vi "Simple Reader.vi"(8 "error in (no error)":errorcluster, 11 "Cryo-Con Driver in":refnum<class "Cryo-Con Driver.lvclass">) -> (0 "error out":errorcluster, 2 "Signals":dbl[](array[numeric]), 3 "Cryo-Con Driver out":refnum<class "Cryo-Con Driver.lvclass">)   [LabVIEW 2019, in "Cryo-Con Driver.lvclass"]
uses:
  Cryo-Con Driver.lvclass
  C:/GitHub/NHMFL_Core/Libraries/Instruments/VISA Instrument/VISA Instrument.lvclass
  C:/GitHub/NHMFL_Core/Libraries/Instruments/Temperature Controller Driver/Temperature Controller Driver.lvclass
  VISA Instrument/VISA Instrument.lvclass/VISA Instrument.ctl
  VISA Instrument/Read VISA resource.vi
  VISA Instrument/Write VISA resource.vi
  Temperature Controller Driver/Read T controller configuration.vi
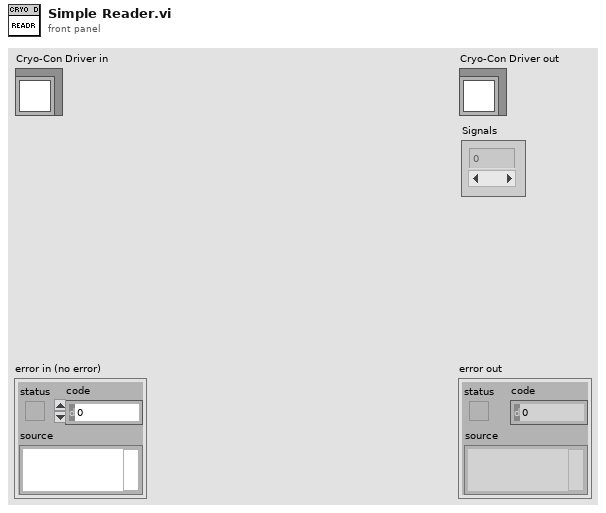
[diagram p1: front panel]
types:
  T1 = typedef "T controller configuration.ctl" = cluster{"Record Channels":string[], "Add raw signal":bool, "New set point":dbl, "Record heater":bool}
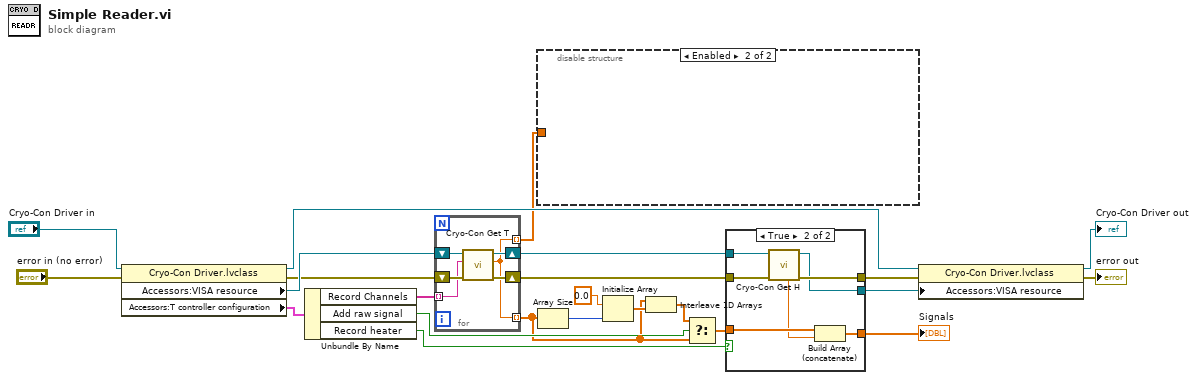
[diagram p0: block diagram]
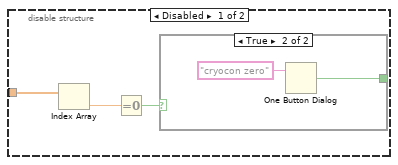
[diagram p2: hidden frame]
diagram:
  n1 = property class="Cryo-Con Driver.lvclass"(reference="Cryo-Con Driver in", error in="error in (no error)") -> (reference out=w17:refnum<class "Cryo-Con Driver.lvclass">, error out=w19:errorcluster, "Accessors:VISA resource"=w20:refnum<visa-resource-name>, "Accessors:T controller configuration"=w21:T1)
  n2 = Unbundle By Name(w21) -> ("Record Channels"=w22:string[], "Add raw signal"=w12:bool, "Record heater"=w4:bool)
  n3 = for {
    tunnel: w22 -> [w25] mode=indexing
    tunnel: [w24] -> w9 mode=indexing
    shift-right: [w27] -> w8
    shift-left: w19 -> [w28]
    shift-right: [w26] -> w7
    shift-left: w20 -> [w29]
    tunnel: [w24] -> w1 mode=indexing
    n4 = call "Cryo-Con Get T.vi"("error in (no error)"=w28, "Channel"=w25, "VISA Resource Name"=w29) -> ("error out"=w27:errorcluster, "Temperature"=w24:dbl, "VISA Resource Name Out"=w26:refnum<visa-resource-name>)  [unwired: 5 in, 1 out]
  }
  n5 = disable-structure shown="Enabled" {
    disable-tunnel: w1 -> [w32 _]
    frame Disabled {
      n6 = Index Array(array=w32) -> (element=w30:dbl)  [unwired: 1 in]
      n7 = Equal To 0?(x=w30) -> (x = 0?=w31:bool)
      n8 = case shown="True" w31 {
        tunnel: [_ w33] -> _
        frame False {
        }
        frame True {
          n9 = One Button Dialog(message="cryocon zero") -> (true=w33:bool)  [unwired: 1 in]
        }
      }
    }
    frame Enabled {
    }
  }
  n10 = Array Size(array=w9) -> (size(s)=w14:i32)
  n11 = Initialize Array(0.0 ("element"), w14) -> (w11:dbl[])
  n12 = Interleave 1D Arrays(w9, w11) -> (w10:dbl[])
  n13 = Select(t=w10, s=w12, f=w9) -> (s? t:f=w3:dbl[])
  n14 = case shown="True" w4 {
    tunnel: w8 -> [w37 w43]
    tunnel: w7 -> [w36 w44]
    tunnel: [w37 w42] -> w6
    tunnel: [w36 w41] -> w5
    tunnel: w3 -> [w35 w40]
    tunnel: [w35 w38] -> w2
    frame False {
    }
    frame True {
      n15 = call "Cryo-Con Get H.vi"("error in (no error)"=w43, "VISA Resource Name"=w44) -> ("error out"=w42:errorcluster, "VISA Resource Name Out"=w41:refnum<visa-resource-name>, "Heat %"=w39:dbl)  [unwired: 6 in, 1 out]
      n16 = Build Array (concatenate)(w40, w39) -> (w38:dbl[])
    }
  }
  "Signals" <- w2
  n17 = property class="Cryo-Con Driver.lvclass"(reference=w17, error in=w6, "Accessors:VISA resource"=w5) -> (reference out=→"Cryo-Con Driver out":refnum<class "Cryo-Con Driver.lvclass">, error out=→"error out":errorcluster)
